vi "JerkConstraint_New.vi"(11 "Max Jerk":dbl format="%20.4f") -> (3 "JERK_CONSTRAINT":T1 {"Max Jerk" format="%20.4f"})   [LabVIEW 2019, in "Trajectory_Library.lvlib"]
doc: "Constructs a centripetal acceleration constraint.\n\nParameters:\n - MaxCentripitalAccel - Maximum Centripetal acceleration (meters/sec^2)\n\nReturns\n - CentripetalAccelConstraint - Constraint data structure."
uses:
  Trajectory_Library.lvlib
  TypeDef/TRAJ_CONSTRAINT_CENTRIPETAL_ACCEL.ctl
  TypeDef/TRAJ_CONSTRAINT_JERK.ctl
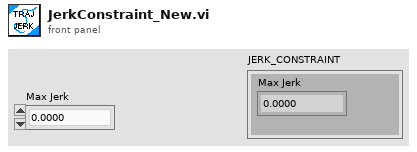
[diagram p1: front panel]
types:
  T1 = typedef "Trajectory_Library.lvlib/TRAJ_CONSTRAINT_JERK.ctl" = cluster{"Max Jerk":dbl}
  T2 = typedef "Trajectory_Library.lvlib/TRAJ_CONSTRAINT_CENTRIPETAL_ACCEL.ctl" = cluster{"Max Cent Accel":dbl}
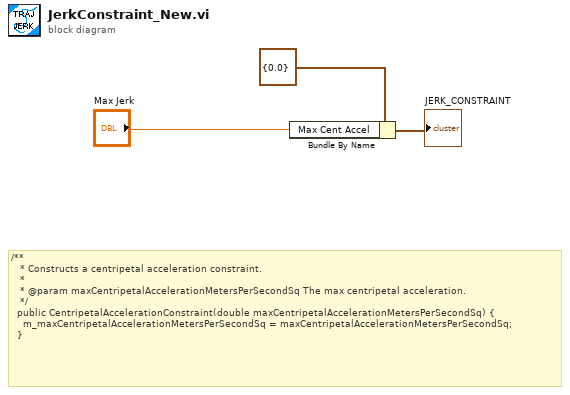
[diagram p0: block diagram]
diagram:
  # "/**\n   * Constructs a centripetal acceleration constraint.\n   *\n   * @param maxCentripetalAccelerationMetersPerSecondSq The max centripetal acceleration.\n   */\n  public CentripetalAccelerationConstraint(double maxCentripetalAccelerationMetersPerSecondSq) {\n    m_maxCentripetalAccelerationMetersPerSecondSq = maxCentripetalAccelerationMetersPerSecondSq;\n  }"
  n1 = Bundle By Name(cluster=T2 {"Max Cent Accel"=0.0} ("CENTRIPETAL_ACCEL_CONSTRAINT"), "Max Cent Accel"="Max Jerk") -> (→"JERK_CONSTRAINT":T2)
